vi "Find Tests from Path.vi"(8 "error in (no error)":errorcluster, 10 "Project or Class Path":path, 11 "Test Case Finder In":refnum<class "Test Finder.lvclass">) -> (0 "error out":errorcluster, 3 "Test Case Finder Out":refnum<class "Test Finder.lvclass">)   [LabVIEW 2020, in "Test Finder.lvclass"]
uses:
  Test Finder.lvclass
  Test Finder.lvclass/Test Finder.ctl
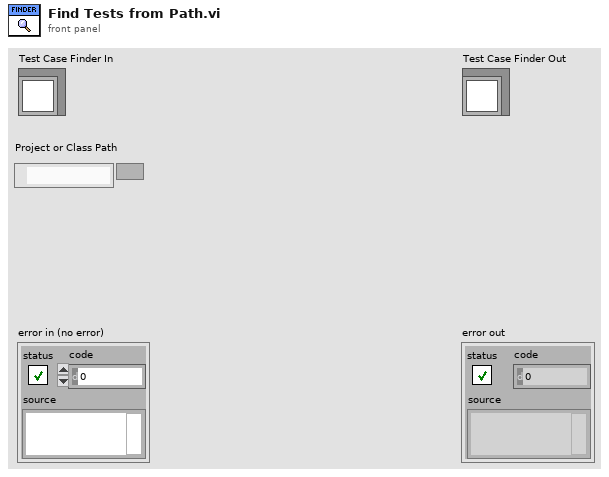
[diagram p1: front panel]
types:
  T1 = cluster{"Inherited Methods":map{string, path}, "Owned Methods":map{string, path}}
  T2 = map{string, cluster{"Inherited Methods":map{string, path}, "Owned Methods":map{string, path}}}
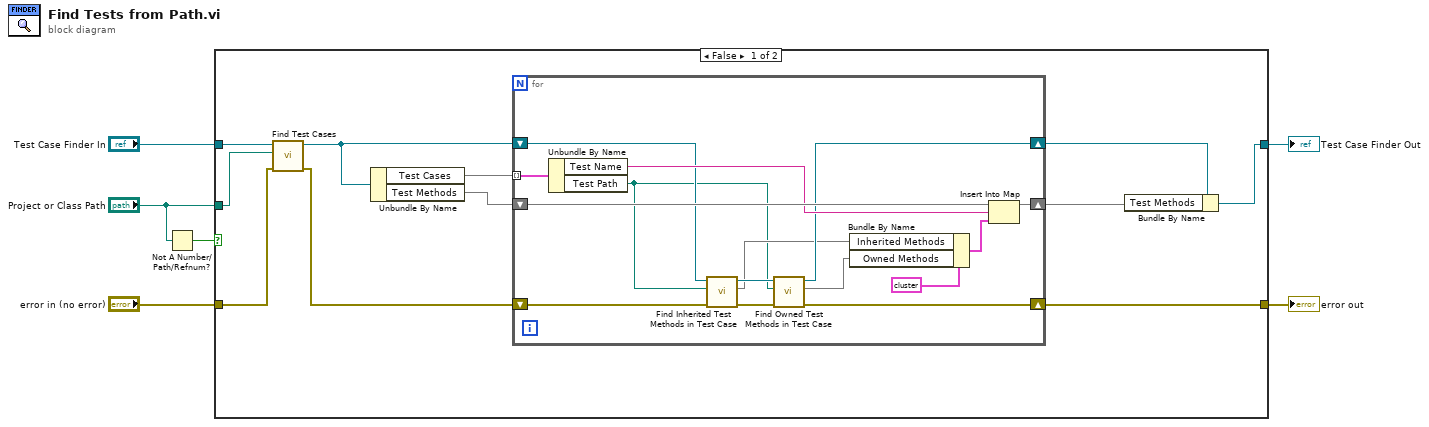
[diagram p0: block diagram]
diagram:
  n1 = Not A Number/Path/Refnum?(number/path/refnum="Project or Class Path") -> (NaN/Path/Refnum?=w1:bool)
  n2 = case shown="False" w1 {
    tunnel: "Test Case Finder In" -> [w17 w34]
    tunnel: [w16 w34] -> w5
    tunnel: "error in (no error)" -> [w14 w33]
    tunnel: [w12 w33] -> w3
    tunnel: "Project or Class Path" -> [w7 _]
    frame False {
      n3 = call-dynamic "Find Test Cases.vi"("error in (no error)"=w14, "Project or Class Path"=w7, "Test Finder In"=w17) -> ("error out"=w13:errorcluster, "Test Finder Out"=w10:refnum<class "Test Finder.lvclass">)  [unwired: 7 in]
      n4 = Unbundle By Name(w10) -> ("Test Cases"=w8:map{string, path}, "Test Methods"=w9:T2)
      n5 = for {
        shift-right: [w24] -> w12
        shift-left: w13 -> [w19]
        shift-right: [w31] -> w15
        shift-left: w9 -> [w32]
        shift-right: [w26] -> w11
        shift-left: w10 -> [w23]
        tunnel: w8 -> [w30] mode=indexing
        n6 = Unbundle By Name(w30) -> ("Test Name"=w29:string, "Test Path"=w20:path)
        n7 = call-dynamic "Find Inherited Test Methods in Test Case.vi"("error in (no error)"=w19, "Test Case Class Path"=w20, "Test Finder In"=w23) -> ("error out"=w18:errorcluster, "Test Methods Out"=w21:map{string, path}, "Test Finder Out"=w22:refnum<class "Test Finder.lvclass">)  [unwired: 6 in]
        n8 = call-dynamic "Find Owned Test Methods in Test Case.vi"("error in (no error)"=w18, "Test Case Class Path"=w20, "Test Finder In"=w22) -> ("error out"=w24:errorcluster, "Test Methods Out"=w25:map{string, path}, "Test Finder Out"=w26:refnum<class "Test Finder.lvclass">)  [unwired: 6 in]
        n9 = Bundle By Name(cluster=T1 {"Inherited Methods"={}, "Owned Methods"={}} ("value"), "Inherited Methods"=w21, "Owned Methods"=w25) -> (w27:T1)
        n10 = Insert Into Map(map in=w32, key=w29, value=w27) -> (map out=w31:T2)  [unwired: 2 out]
      }
      n11 = Bundle By Name(cluster=w11, "Test Methods"=w15) -> (w16:refnum<class "Test Finder.lvclass">)
    }
    frame True {
    }
  }
  "error out" <- w3
  "Test Case Finder Out" <- w5
